vi "Load Config.vi"(8 "error in (no error)":errorcluster, 11 "Target Folder":path) -> (0 "error out":errorcluster, 3 "Config":T1={"Main"={"Menu Folder"="", "Re-Create Menu Folder?"=FALSE, "Allow mnu replace?"=FALSE}, "File Filter"={"Exclude Prefixes"=[], "Ignore Names"=[], "Include Extensions"=[], "Exclude Postfixes"=[]}, "Folder Filter"={"Exclude Prefixes"=[], "Ignore Names"=[]}, "File Name Edit"={"Pre Split String"="", "Post Split String"=""}, "Folder Name Edit"={"Pre Split String"="", "Post Split String"="", "Deletion Strings"=[]}, "Folder Icon Map"={}, "Default Palette Data"={"Display Name Override"="", "View Format"=2, "Palette Width"=0, "Help Tag"="", "Help File Path"=path "", "Palette Description"=""}, "Default File Data"={"Display Name Override"="", "Place VI Contents?"=FALSE}, "Palette Override map"={}, "File Override map"={}} {"Default Palette Data"."View Format" items=["Icons", "Text", "Icons and Text"]})   [LabVIEW 2019, in "AutoMenuCreator.lvlib"]
doc: "Load data from the AutoMenu Config.ini if it exists, create it if it doesn't before loading. Creation is handled by creating a copy of the 'Menu Config Template.ini'-file."
uses:
  AutoMenuCreator.lvlib
  Ctl/Ctl_Config.ctl
  Ctl/Ctl_Config_Main.ctl
  Ctl/Ctl_Config_File Filter.ctl
  Ctl/Ctl_Config_Folder Filter.ctl
  Ctl/Ctl_Config_File Name Edit.ctl
  Ctl/Ctl_Config_Folder Name Edit.ctl
  Ctl/Ctl_Config_Folder Icon Map.ctl
  Ctl/Ctl_Config_Palette Data.ctl
  <vilib>/Palette API/Palette Menu/Public Type Define/View Format.ctl
  Ctl/Ctl_Config_File Data.ctl
  <vilib>/Utility/config.llb/NI_LVConfig.lvlib
  <vilib>/Palette API/Palette Menu/Palette Menu.lvlib
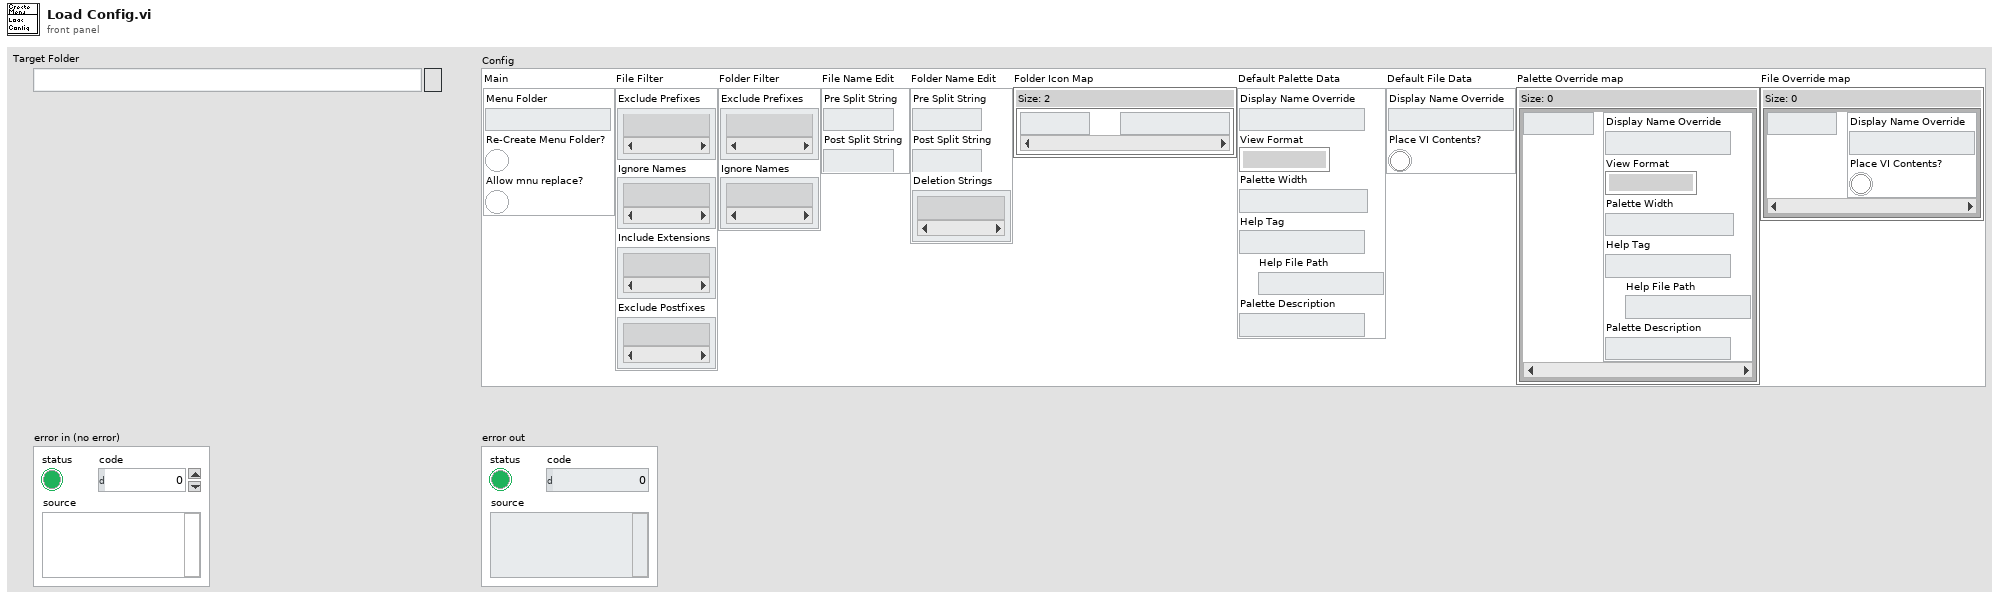
[diagram p1: front panel]
types:
  T1 = typedef "AutoMenuCreator.lvlib/Ctl_Config.ctl" = cluster{"Main":T2, "File Filter":T3, "Folder Filter":T4, "File Name Edit":T5, "Folder Name Edit":T6, "Folder Icon Map":T7, "Default Palette Data":T8, "Default File Data":T10, "Palette Override map":map{string, T8}, "File Override map":map{string, T10}}
  T2 = typedef "AutoMenuCreator.lvlib/Ctl_Config_Main.ctl" = cluster{"Menu Folder":string, "Re-Create Menu Folder?":bool, "Allow mnu replace?":bool}
  T3 = typedef "AutoMenuCreator.lvlib/Ctl_Config_File Filter.ctl" = cluster{"Exclude Prefixes":string[], "Ignore Names":string[], "Include Extensions":string[], "Exclude Postfixes":string[]}
  T4 = typedef "AutoMenuCreator.lvlib/Ctl_Config_Folder Filter.ctl" = cluster{"Exclude Prefixes":string[], "Ignore Names":string[]}
  T5 = typedef "AutoMenuCreator.lvlib/Ctl_Config_File Name Edit.ctl" = cluster{"Pre Split String":string, "Post Split String":string}
  T6 = typedef "AutoMenuCreator.lvlib/Ctl_Config_Folder Name Edit.ctl" = cluster{"Pre Split String":string, "Post Split String":string, "Deletion Strings":string[]}
  T7 = typedef "AutoMenuCreator.lvlib/Ctl_Config_Folder Icon Map.ctl" = map{string, path}
  T8 = typedef "AutoMenuCreator.lvlib/Ctl_Config_Palette Data.ctl" = cluster{"Display Name Override":string, "View Format":T9, "Palette Width":i16, "Help Tag":string, "Help File Path":path, "Palette Description":string}
  T9 = typedef "Palette Menu.lvlib/View Format.ctl" = u16
  T10 = typedef "AutoMenuCreator.lvlib/Ctl_Config_File Data.ctl" = cluster{"Display Name Override":string, "Place VI Contents?":bool}
  T11 = typedef "NI_LVConfig.lvlib/Config Data RefNum.ctl" = refnum<k1>
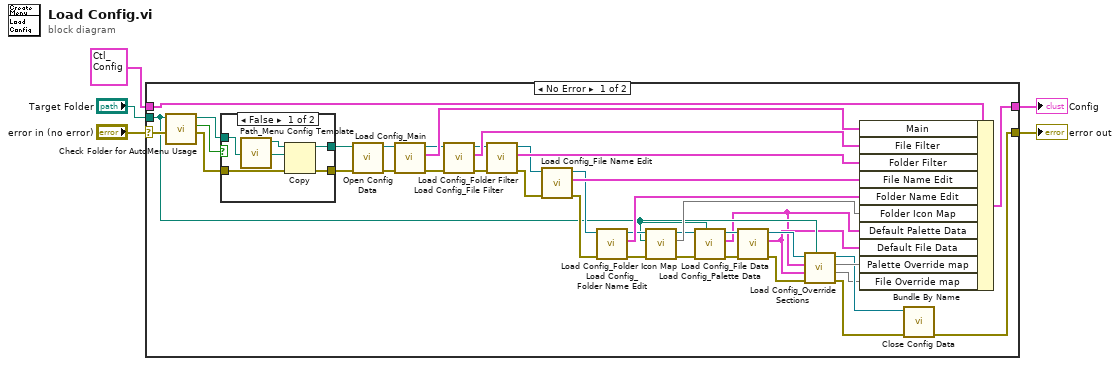
[diagram p0: block diagram]
diagram:
  n1 = case shown="No Error" "error in (no error)" {
    selector: "error in (no error)" -> [w18 w53]
    tunnel: "Target Folder" -> [w9 _]
    tunnel: [w40 w53] -> w3
    tunnel: T1 {"Main"={"Menu Folder"="", "Re-Create Menu Folder?"=FALSE, "Allow mnu replace?"=FALSE}, "File Filter"={"Exclude Prefixes"=[], "Ignore Names"=[], "Include Extensions"=[], "Exclude Postfixes"=[]}, "Folder Filter"={"Exclude Prefixes"=[], "Ignore Names"=[]}, "File Name Edit"={"Pre Split String"="", "Post Split String"=""}, "Folder Name Edit"={"Pre Split String"="", "Post Split String"="", "Deletion Strings"=[]}, "Folder Icon Map"={}, "Default Palette Data"={"Display Name Override"="", "View Format"=2, "Palette Width"=0, "Help Tag"="", "Help File Path"=path "", "Palette Description"=""}, "Default File Data"={"Display Name Override"="", "Place VI Contents?"=FALSE}, "Palette Override map"={}, "File Override map"={}} ("Config") -> [w37 w52]
    tunnel: [w36 w52] -> w1
    frame No Error {
      n2 = call "Check Folder for AutoMenu Usage.vi"("Target"=w9) -> ("Uses AutoMenu?"=w44:bool, "Found AutoMenu Config.ini path"=w43:path)  [unwired: 9 in]
      n3 = case shown="False" w44 {
        tunnel: w43 -> [w48 w51]
        tunnel: [w46 w51] -> w42
        tunnel: w18 -> [w47 w50]
        tunnel: [w45 w50] -> w41
        frame False {
          n4 = call "Path_Menu Config Template.vi"() -> ("Menu Config Template path"=w49:path)  [unwired: 11 in]
          n5 = Copy(8:w47, 10:w48, 11:w49) -> (0:w45:errorcluster, 3:w46:path)  [unwired: 2 in, 1 out]
        }
        frame True {
        }
      }
      n6 = call <vilib>:"Open Config Data.vi"("error in (no error)"=w41, "configuration file path"=w42) -> ("error out"=w38:errorcluster, "refnum"=w39:T11)  [unwired: 7 in, 1 out]
      n7 = call "Load Config_Main.vi"("error in (no error)"=w38, "Refnum in"=w39) -> ("error out"=w33:errorcluster, "Main"=w35:T2, "Refnum out"=w34:T11)  [unwired: 7 in]
      n8 = call "Load Config_File Filter.vi"("error in (no error)"=w33, "Refnum in"=w34) -> ("error out"=w32:errorcluster, "File Filter"=w31:T3, "Refnum out"=w29:T11)  [unwired: 7 in]
      n9 = call "Load Config_Folder Filter.vi"("error in (no error)"=w32, "Refnum in"=w29) -> ("error out"=w30:errorcluster, "Folder Filter"=w28:T4, "Refnum out"=w26:T11)  [unwired: 7 in]
      n10 = call "Load Config_File Name Edit.vi"("error in (no error)"=w30, "Refnum in"=w26) -> ("error out"=w27:errorcluster, "File Name Edit"=w25:T5, "Refnum out"=w23:T11)  [unwired: 7 in]
      n11 = call "Load Config_Folder Name Edit.vi"("error in (no error)"=w27, "Refnum in"=w23) -> ("error out"=w24:errorcluster, "Folder Name Edit"=w22:T6, "Refnum out"=w20:T11)  [unwired: 7 in]
      n12 = call "Load Config_Folder Icon Map.vi"("error in (no error)"=w24, "Target Folder"=w9, "Refnum in"=w20) -> ("error out"=w21:errorcluster, "Folder Icon Map"=w19:T7, "Refnum out"=w16:T11)  [unwired: 6 in]
      n13 = call "Load Config_Palette Data.vi"("Target Folder"=w9, "error in (no error)"=w21, "Refnum in"=w16) -> ("error out"=w17:errorcluster, "Palette Data out"=w6:T8, "Refnum out"=w15:T11)  [unwired: 6 in]
      n14 = call "Load Config_File Data.vi"("error in (no error)"=w17, "Refnum in"=w15) -> ("error out"=w14:errorcluster, "File Data out"=w7:T10, "Refnum out"=w11:T11)  [unwired: 7 in]
      n15 = call "Load Config_Override Sections.vi"("Target Folder"=w9, "error in (no error)"=w14, "Default File Data"=w7, "Default Palette Data"=w6, "Refnum in"=w11) -> ("error out"=w13:errorcluster, "File Override map"=w8:map{string, T10}, "Palette Override map"=w12:map{string, T8}, "Refnum out"=w10:T11)  [unwired: 3 in]
      n16 = Bundle By Name(cluster=w37, "Main"=w35, "File Filter"=w31, "Folder Filter"=w28, "File Name Edit"=w25, "Folder Name Edit"=w22, "Folder Icon Map"=w19, "Default Palette Data"=w6, "Default File Data"=w7, "Palette Override map"=w12, "File Override map"=w8) -> (w36:T1)
      n17 = call <vilib>:"Close Config Data.vi"("error in (no error)"=w13, "refnum"=w10) -> ("error out"=w40:errorcluster)  [unwired: 8 in, 1 out]
    }
    frame Error {
    }
  }
  "error out" <- w3
  "Config" <- w1
